vi "Write Status.vi"(8 "error in (no error)":errorcluster, 10 "Status":bool, 11 "SimFlatShutt in":refnum<class "SimFlatShutt.lvclass">) -> (0 "error out":errorcluster, 3 "SimFlatShutt out":refnum<class "SimFlatShutt.lvclass">)   [LabVIEW 2016, in "SimFlatShutt.lvclass"]
uses:
  SimFlatShutt.lvclass
  Shutter.lvclass
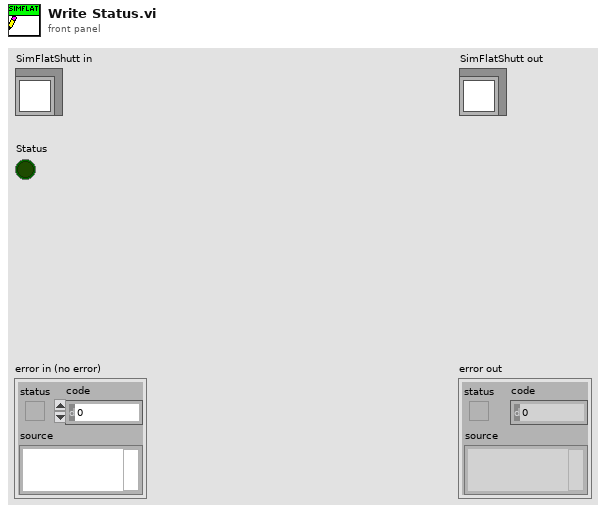
[diagram p1: front panel]
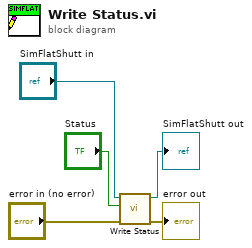
[diagram p0: block diagram]
diagram:
  n1 = call-parent "Write Status.vi"("error in (no error)"="error in (no error)", "Status"="Status", "Shutter in"="SimFlatShutt in") -> ("error out"=→"error out":errorcluster, "Shutter out"=→"SimFlatShutt out":refnum<class "SimFlatShutt.lvclass">)  [unwired: 7 in]
